vi "bodyTest.vi"(7 "LabVIEW Web Service Request":refnum<class "Web Request.lvclass">, 10 "nominalPressure":dbl caption="pressure" format="%#g", 11 "time":dbl format="%#g") -> (3 "Current Pressure Pressure":dbl)   [LabVIEW 2015]
uses:
  <vilib>/wsapi/Web Request.lvclass
  <vilib>/Waveform/WDTOps.llb/WDT Append Waveforms DBL.vi
panel:
  out "value":string
  in  "Start timer":bool
  out "data":waveform(dbl)[](graph)
  out "timer":dbl
  in  "Stop timer":bool
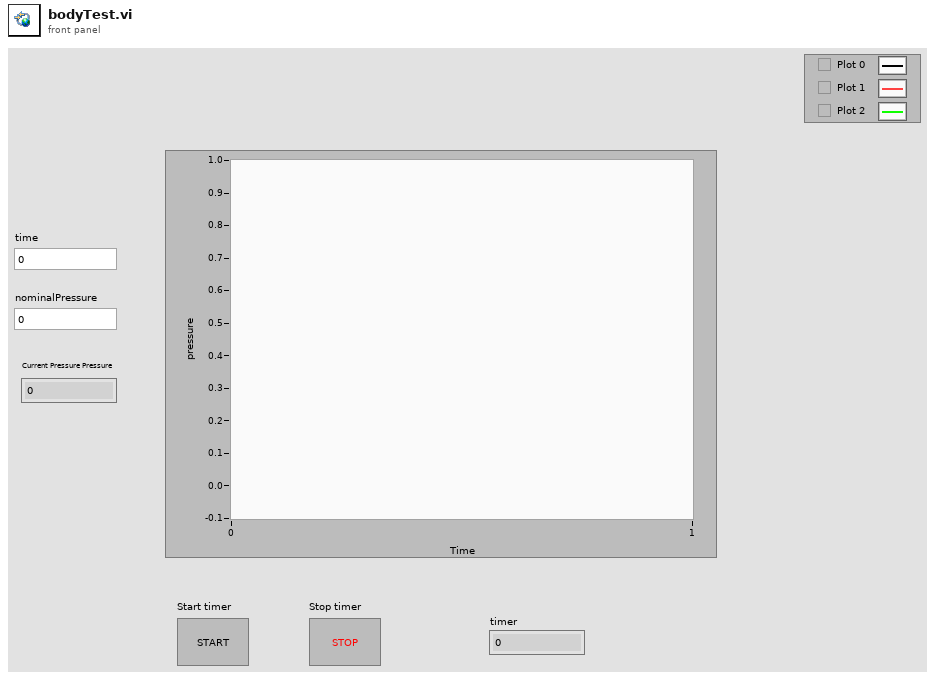
[diagram p1: front panel]
types:
  T1 = typedef "imagedata.ctl" = cluster{"image type":i32, "image depth":i32, "image":u8[], "mask":u8[], "colors":u32[], "Rectangle":cluster{"left":i16, "top":i16, "right":i16, "bottom":i16}}
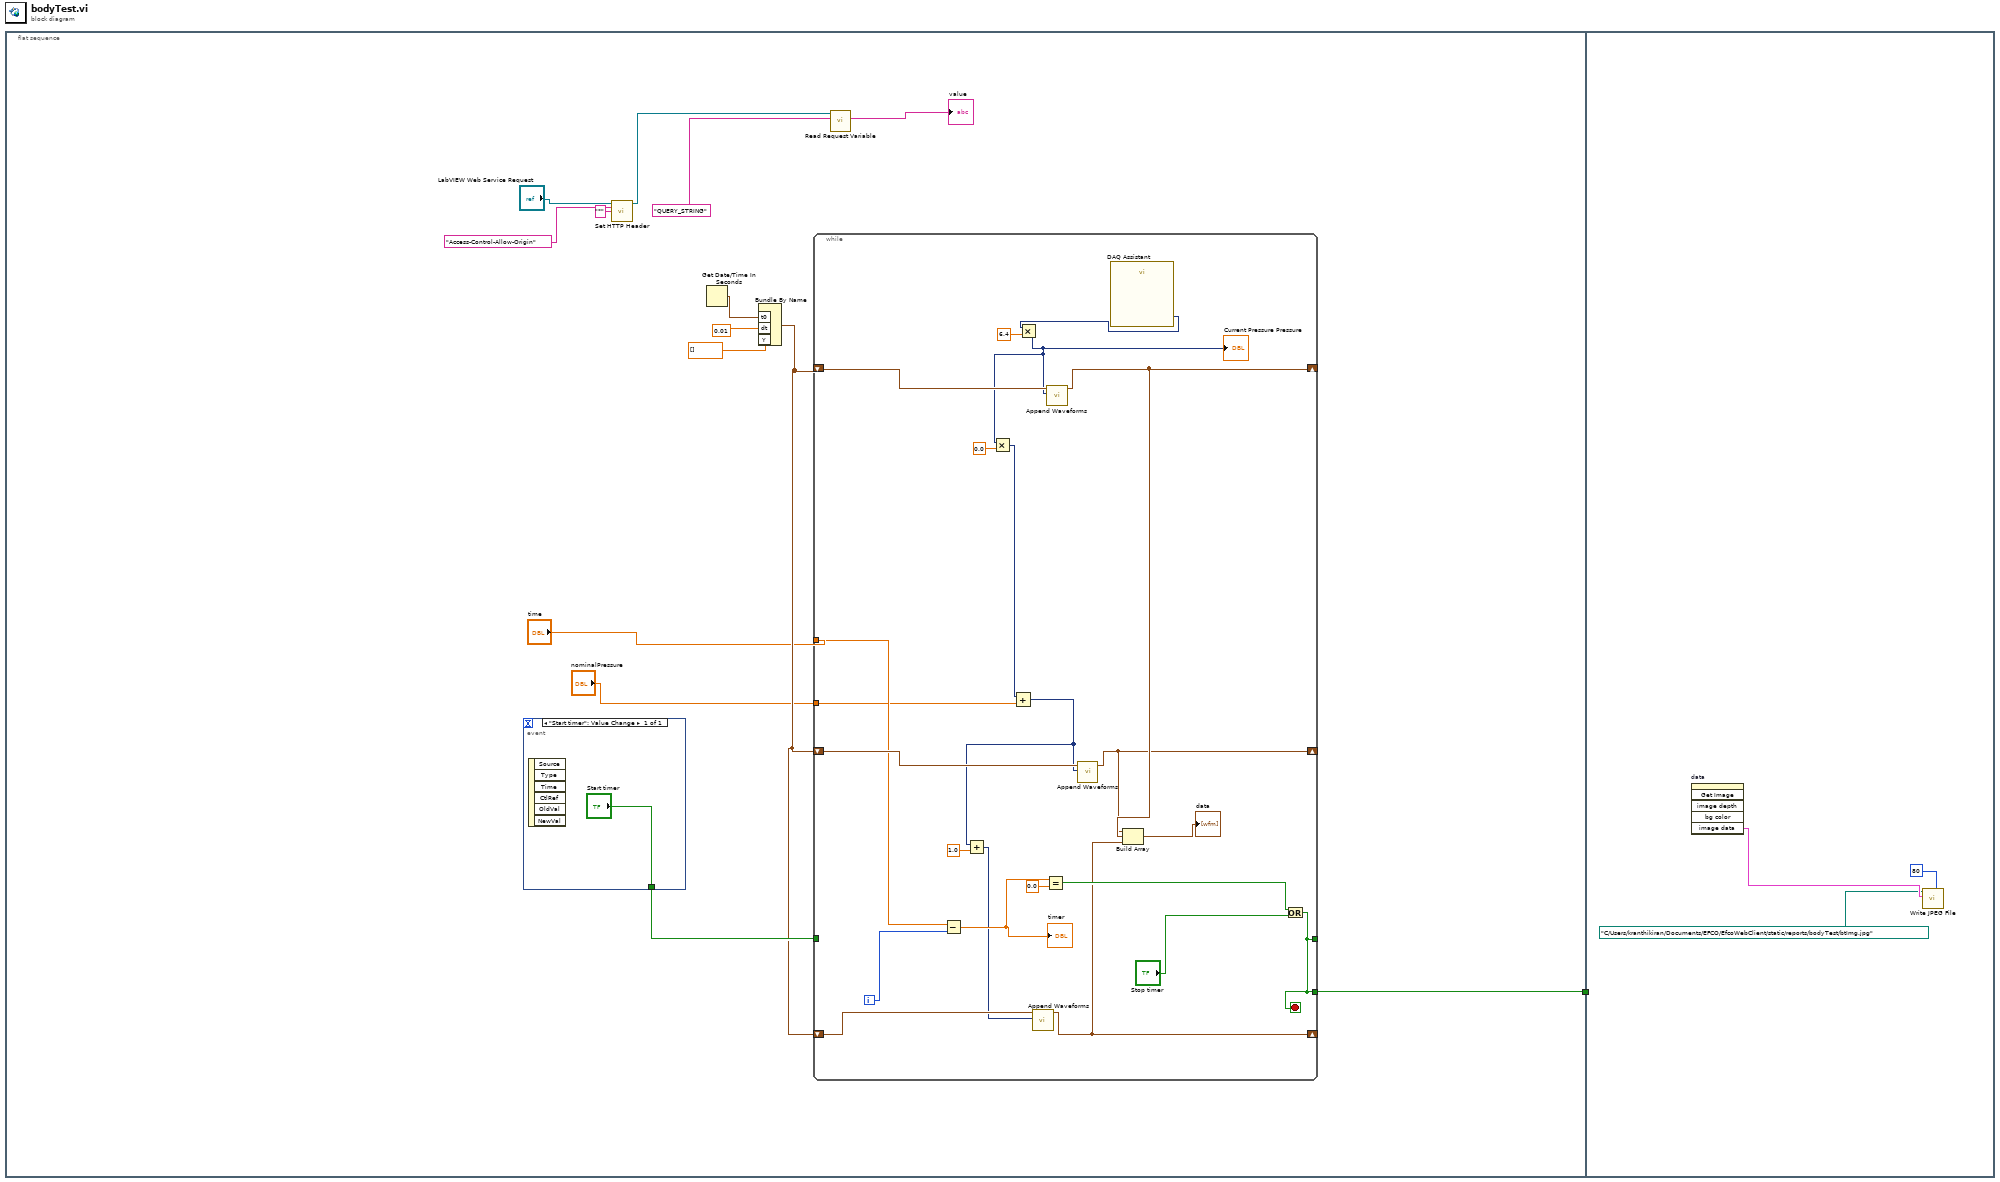
[diagram p0: block diagram]
diagram:
  n1 = flat-sequence {
    tunnel: [w2] -> w1
    tunnel: w1 -> [_]
    frame #0 {
      n2 = event shown="[0] \"Start timer\": Value Change" {
        selector: _ -> [_]
        dyn-events: _ -> [_]
        timeout: _ -> [_]
        tunnel: ["Start timer"] -> w12
        event "Start timer": Value Change {
          n3 = event-data() -> ()  [unwired: 1 in, 6 out]
        }
      }
      n4 = call <vilib>:"Set HTTP Header.vi"("LabVIEW Web Service Request"="LabVIEW Web Service Request", "header"="Access-Control-Allow-Origin", "header value"="*") -> ("LabVIEW Web Service Request out"=w5:refnum<class "Web Request.lvclass">)  [unwired: 11 in, 1 out]
      n5 = Get Date/Time In Seconds() -> (seconds since 1Jan1904=w15:timestamp)
      n6 = Bundle By Name("t0"=w15, "dt"=0.01, "Y"=dbl[] []) -> (w11:waveform(dbl))  [unwired: 1 in]
      n7 = while {
        shift-right: [w33] -> _
        shift-left: w11 -> [w39]
        tunnel: "time" -> [w28]
        shift-right: [w32] -> _
        shift-left: w11 -> [w37]
        tunnel: w12 -> [_]
        shift-right: [w19] -> _
        shift-left: w11 -> [w23]
        tunnel: "nominalPressure" -> [w18]
        tunnel: [w17] -> _
        tunnel: [w17] -> w2
        i -> [w29]
        stop <- w17 stop-if-true
        n8 = Subtract(x=w28, y=w29) -> (x-y=w27:dbl)
        "timer" <- w27
        n9 = Equal?(x=w27, y=0.0) -> (x = y?=w25:bool)
        n10 = call "DAQ Assistant"() -> ("data"=w31:dynamicdata)  [unwired: 16 in, 3 out]
        n11 = Multiply(x=w31, y=6.4) -> (x*y=w36:dynamicdata)
        "Current Pressure Pressure" <- w36
        n12 = Multiply(x=w36, y=0.0) -> (x*y=w34:dynamicdata)
        n13 = Add(x=w34, y=w18) -> (x+y=w22:dynamicdata)
        n14 = Add(x=w22, y=1.0) -> (x+y=w20:dynamicdata)
        n15 = call-poly <vilib>:"Append Waveforms.vi"("waveform B"=w20, "waveform A"=w23) -> ("waveform out"=w19:waveform(dbl))  [unwired: 8 in, 1 out]
        n16 = call-poly <vilib>:"Append Waveforms.vi"("waveform B"=w36, "waveform A"=w39) -> ("waveform out"=w33:waveform(dbl))  [unwired: 8 in, 1 out]
        n17 = call-poly <vilib>:"Append Waveforms.vi"("waveform B"=w22, "waveform A"=w37) -> ("waveform out"=w32:waveform(dbl))  [unwired: 8 in, 1 out]
        n18 = Build Array(w32, w33, w19) -> (→"data":waveform(dbl)[])
        n19 = Or(x=w25, y="Stop timer") -> (x .or. y?=w17:bool)
      }
      n20 = call <vilib>:"Read Request Variable.vi"("LabVIEW Web Service Request"=w5, "variable name"="QUERY_STRING") -> ("value"=→"value":string)  [unwired: 11 in, 2 out]
    }
    frame #1 {
      n21 = invoke on="data" class="WFGraph (strict)" method="Get Image"() -> ("image data"=w42:T1)  [unwired: 6 in, 5 out]
      n22 = call <vilib>:"Write JPEG File.vi"("quality (80)"=80, "image data"=w42, "path to JPEG file"=path "C:/Users/kranthikiran/Documents/EFCO/EfcoWebClient/static/reports/bodyTest/btImg.jpg") -> ()  [unwired: 7 in, 2 out]
    }
  }
